vi "Initialize.vi"(0 "BaseProducer in":refnum<class "BaseProducer.lvclass">, 1 "connection information":string, 2 "test state file path":path, 5 "table":string, 7 "columns":string[](array[string]), 9 "IO Task Cluster":T1={"Dynamic P Tasks"="DynP_all_S6AI0-4", "AI Tasks"="AiTasks_TC_P_S3", "DIO Tasks"="MFCOutputEnable_S2P0L67", "AO Tasks"="MFCVoltageOut_S2AO0-3"}, 11 "error in (no error)":errorcluster, 12 "Username":string, 13 "Password":string) -> (4 "BaseProducer out":refnum<class "BaseProducer.lvclass">, 15 "error out":errorcluster)   [LabVIEW 2013, in "BaseProducer.lvclass"]
doc: "This method initializes the producer, setting data element values, opening data files, etc. It does NOT start IO tasks. Note that this method will do nothing if the object has already been initialized. This is to avoid spawning mulitple data write processes."
uses:
  BaseProducer.lvclass
  IO Task Cluster.ctl
  BaseProducer.lvclass/BaseProducer.ctl
  DbMeasurement/DbMeasurement.lvclass
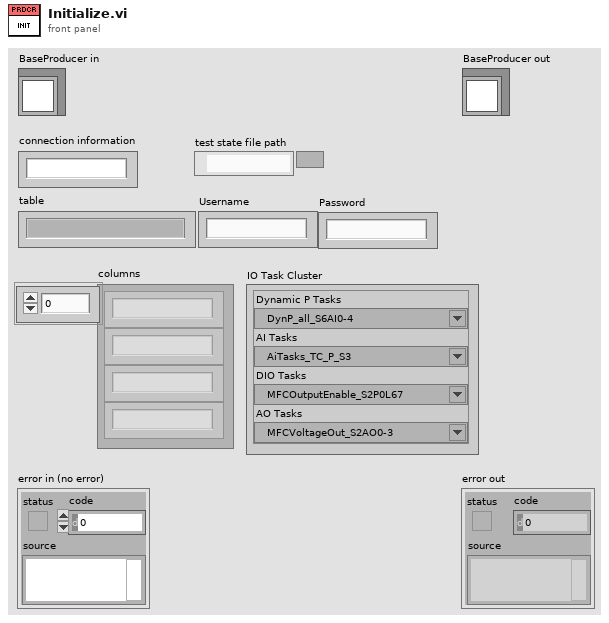
[diagram p1: front panel]
types:
  T1 = typedef "BaseProducer.lvclass/IO Task Cluster.ctl" = cluster{"Dynamic P Tasks":refnum<k21>, "AI Tasks":refnum<k21>, "DIO Tasks":refnum<k21>, "AO Tasks":refnum<k21>}
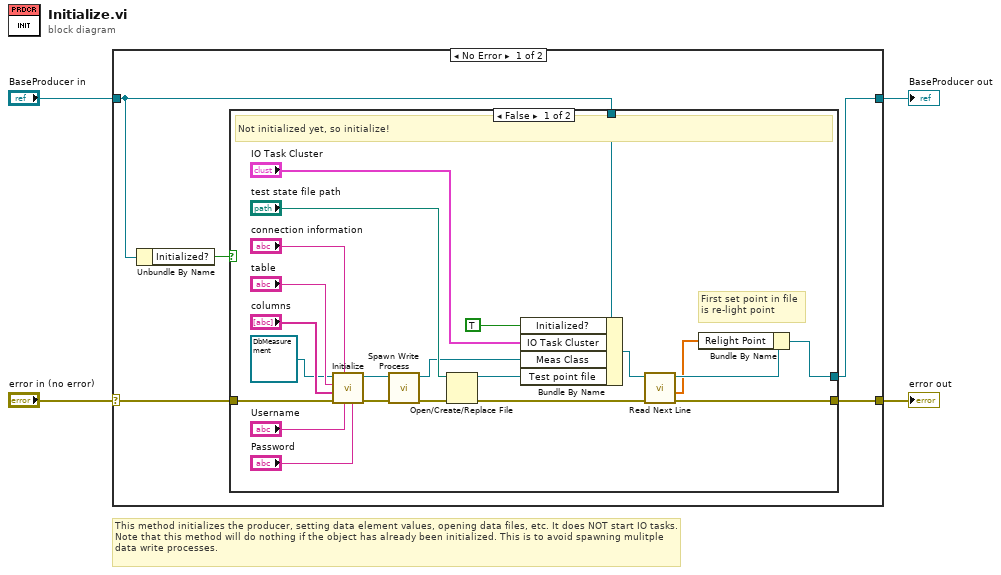
[diagram p0: block diagram]
diagram:
  # "This method initializes the producer, setting data element values, opening data files, etc. It does NOT start IO tasks. Note that this method will do nothing if the object has already been initialized. This is to avoid spawning mulitple data write processes."
  n1 = case shown="No Error" "error in (no error)" {
    selector: "error in (no error)" -> [w9 w35]
    tunnel: [w8 w35] -> w3
    tunnel: [w5 w34] -> w1
    tunnel: "BaseProducer in" -> [w7 w34]
    frame No Error {
      n2 = Unbundle By Name(w7) -> ("Initialized?"=w6:bool)
      n3 = case shown="False" w6 {
        tunnel: w9 -> [w31 w33]
        tunnel: [w17 w33] -> w8
        tunnel: w7 -> [w22 w32]
        tunnel: [w16 w32] -> w5
        frame False {
          # "First set point in file\nis re-light point"
          # "Not initialized yet, so initialize!"
          n4 = call "Initialize.vi"("Password"="Password", "Username"="Username", "connection information"="connection information", "error in (no error)"=w31, "columns"="columns", "table"="table", "DbMeasurement in"=refnum<class "DbMeasurement.lvclass"> refnum ("DbMeasurement.lvclass")) -> ("error out"=w28:errorcluster, "DbMeasurement out"=w27:refnum<class "DbMeasurement.lvclass">)  [unwired: 3 in]
          n5 = call "Spawn Write Process.vi"("error in (no error)"=w28, "DbMeasurement in"=w27) -> ("error out"=w26:errorcluster, "DbMeasurement out"=w21:refnum<class "DbMeasurement.lvclass">)  [unwired: 8 in]
          n6 = Open/Create/Replace File(file path (use dialog)="test state file path", error in=w26) -> (refnum out=w24:refnum<file>, error out=w13:errorcluster)  [unwired: 4 in, 1 out]
          n7 = Bundle By Name(cluster=w22, "Initialized?"=TRUE, "IO Task Cluster"="IO Task Cluster", "Meas Class"=w21, "Test point file"=w24) -> (w14:refnum<class "BaseProducer.lvclass">)
          n8 = call "Read Next Line.vi"("error in (no error)"=w13, "BaseProducer in"=w14) -> ("error out"=w17:errorcluster, "Operating Point"=w15:dbl[], "BaseProducer out"=w18:refnum<class "BaseProducer.lvclass">)  [unwired: 6 in, 1 out]
          n9 = Bundle By Name(cluster=w18, "Relight Point"=w15) -> (w16:refnum<class "BaseProducer.lvclass">)
        }
        frame True {
          # "Already initialized. Do nothing!"
        }
      }
    }
    frame Error {
    }
  }
  "error out" <- w3
  "BaseProducer out" <- w1
